vi "EventLoopForStatus.vi"(8 "error in (no error)":errorcluster, 9 "Event Registration Refnum":refnum<event-registration>, 10 "Events":T1, 11 "MulticolumnListbox in":refnum<vi>) -> (0 "error out":errorcluster)   [LabVIEW 2020, in "SolutionBuilder.lvlib"]
uses:
  SolutionBuilder/SolutionBuilder.lvlib
  SolutionBuilder/Events.ctl
  SolutionBuilder/EventUpdateList.ctl
  SolutionBuilder/EventItemBuilt.ctl
  SolutionBuilder/SolutionBuilder.lvclass
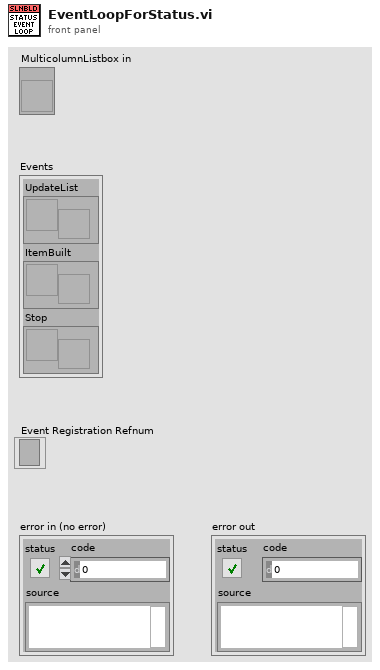
[diagram p1: front panel]
types:
  T1 = typedef "SolutionBuilder.lvlib/Events.ctl" = cluster{"UpdateList":T2, "ItemBuilt":T3, "Stop":refnum<user-event>}
  T2 = typedef "SolutionBuilder.lvlib/SolutionBuilder.lvclass/EventUpdateList.ctl" = refnum<user-event>
  T3 = typedef "SolutionBuilder.lvlib/SolutionBuilder.lvclass/EventItemBuilt.ctl" = refnum<user-event>
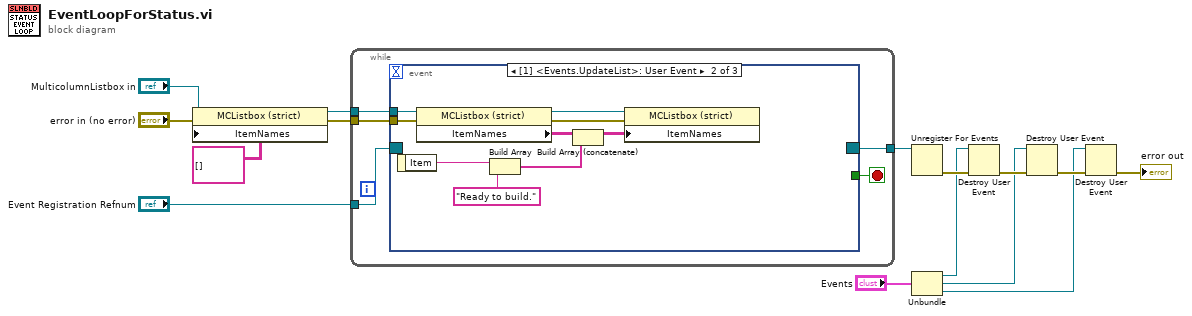
[diagram p0: block diagram]
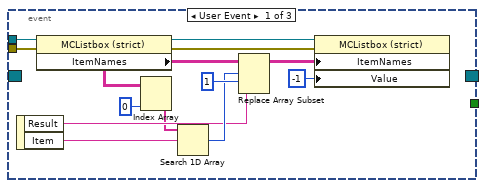
[diagram p2: hidden frame]
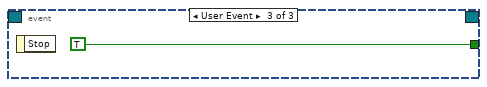
[diagram p3: hidden frame]
diagram:
  n1 = property class="MCListbox (strict)"(reference="MulticolumnListbox in", error in="error in (no error)", "ItemNames"=string[][] [] ("Item Names")) -> (reference out=w7:refnum<vi>, error out=w2:errorcluster)
  n2 = while {
    tunnel: w2 -> [w20]
    tunnel: "Event Registration Refnum" -> [w19]
    tunnel: w7 -> [w17]
    tunnel: [w16] -> w13
    stop <- w18 stop-if-true
    n3 = event shown="[1] <Events.UpdateList>: User Event" {
      selector: w19 -> [_ _ _]
      dyn-events: [_ _ _] -> w16
      timeout: _ -> [_ _ _]
      tunnel: w20 -> [w30 w42 _]
      tunnel: [_ _ TRUE] -> w18
      tunnel: w17 -> [w31 w41 _]
      event User Event {
        n4 = event-data() -> ("Result"=w25:string, "Item"=w26:string)  [unwired: 1 in]
        n5 = property class="MCListbox (strict)"(reference=w31, error in=w30) -> (reference out=w29:refnum<vi>, error out=w28:errorcluster, "ItemNames"=w24:string[][])
        n6 = Index Array(array=w24, index (col)=0 ("disabled index (col)")) -> (element=w22:string[])  [unwired: 1 in]
        n7 = Search 1D Array(1D array=w22, element=w26) -> (index of element=w32:i32)  [unwired: 1 in]
        n8 = Replace Array Subset(array=w24, new element=w25, index (row)=w32, index (col)=1 ("disabled index (col)")) -> (w27:string[][])
        n9 = property class="MCListbox (strict)"(reference=w29, error in=w28, "ItemNames"=w27, "Value"=-1) -> ()  [unwired: 2 out]
      }
      event User Event {
        n10 = event-data() -> ("Item"=w34:string)  [unwired: 1 in]
        n11 = property class="MCListbox (strict)"(reference=w41, error in=w42) -> (reference out=w35:refnum<vi>, error out=w36:errorcluster, "ItemNames"=w40:string[][])
        n12 = Build Array(w34, "Ready to build." ("element")) -> (w38:string[])
        n13 = Build Array (concatenate)(w40, w38) -> (w37:string[][])
        n14 = property class="MCListbox (strict)"(reference=w35, error in=w36, "ItemNames"=w37) -> ()  [unwired: 2 out]
      }
      event User Event {
        n15 = event-data() -> ()  [unwired: 1 in, 1 out]
      }
    }
  }
  n16 = Unregister For Events(event registration refnum=w13) -> (error out=w14:errorcluster)  [unwired: 1 in]
  n17 = Unbundle("Events") -> ("UpdateList"=w4:T2, "ItemBuilt"=w3:T3, "Stop"=w5:refnum<user-event>)
  n18 = Destroy User Event(user event=w4, error in=w14) -> (error out=w15:errorcluster)
  n19 = Destroy User Event(user event=w3, error in=w15) -> (error out=w12:errorcluster)
  n20 = Destroy User Event(user event=w5, error in=w12) -> (error out=→"error out":errorcluster)
